vi "MotionProfileGenerator2.vi"(1 "MotionProfileGeneratorParameters":T1={"Trajectory Point Interval (ms)"=10, "Maximum Travel Speed (units/s)"=0.0, "Velocity Ramp Time (ms)"=0.0, "Acceleration Ramp Time (ms)"=1.0} {"Acceleration Ramp Time (ms)" min=1.0; "Velocity Ramp Time (ms)" min=1.0; "Maximum Travel Speed (units/s)" min=0.0; "Trajectory Point Interval (ms)" items=["TrajectoryDuration_0ms"=0, "TrajectoryDuration_5ms"=5, "TrajectoryDuration_10ms"=10, "TrajectoryDuration_20ms"=20, "TrajectoryDuration_30ms"=30, "TrajectoryDuration_40ms"=40, "TrajectoryDuration_50ms"=50, "TrajectoryDuration_100ms"=100]}, 2 "Starting Position (units)":dbl, 3 "Travel Distance (units)":dbl) -> (0 "Trajectory Points":T3[](array[typedef]) {"Time (ms)" items=["TrajectoryDuration_0ms"=0, "TrajectoryDuration_5ms"=5, "TrajectoryDuration_10ms"=10, "TrajectoryDuration_20ms"=20, "TrajectoryDuration_30ms"=30, "TrajectoryDuration_40ms"=40, "TrajectoryDuration_50ms"=50, "TrajectoryDuration_100ms"=100]})   [LabVIEW 2018, in "ArgosLib.lvlib"]
uses:
  ArgosLib.lvlib
  TypeDefs/TrajectoryPoint.ctl
  <vilib>/Rock Robotics/WPI/ThirdParty/Phoenix-LabVIEW/Motor Controller/Controls/CTRE_Phoenix_MotorControl_TrajectoryPointTimeDur.ctl
  TypeDefs/MotionProfileGeneratorParams.ctl
panel:
  out "Input":bool
  out "T4":dbl
  out "fl2":dbl
  out "fl1":dbl
  out "n":dbl
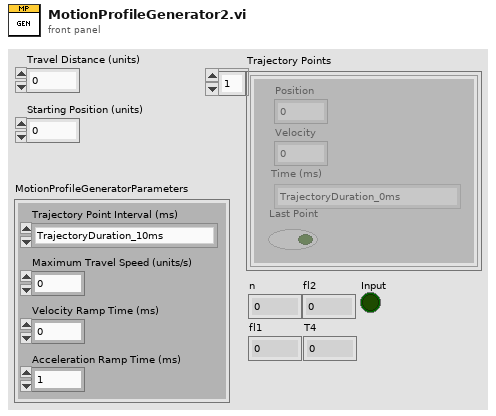
[diagram p1: front panel]
types:
  T1 = typedef "ArgosLib.lvlib/MotionProfileGeneratorParams.ctl" = cluster{"Trajectory Point Interval (ms)":T2, "Maximum Travel Speed (units/s)":dbl, "Velocity Ramp Time (ms)":dbl, "Acceleration Ramp Time (ms)":dbl}
  T2 = typedef "CTRE_Phoenix_MotorControl_TrajectoryPointTimeDur.ctl" = i32
  T3 = typedef "ArgosLib.lvlib/TrajectoryPoint.ctl" = cluster{"Position ":dbl, "Velocity ":dbl, "Time (ms)":T2, "Last Point":bool}
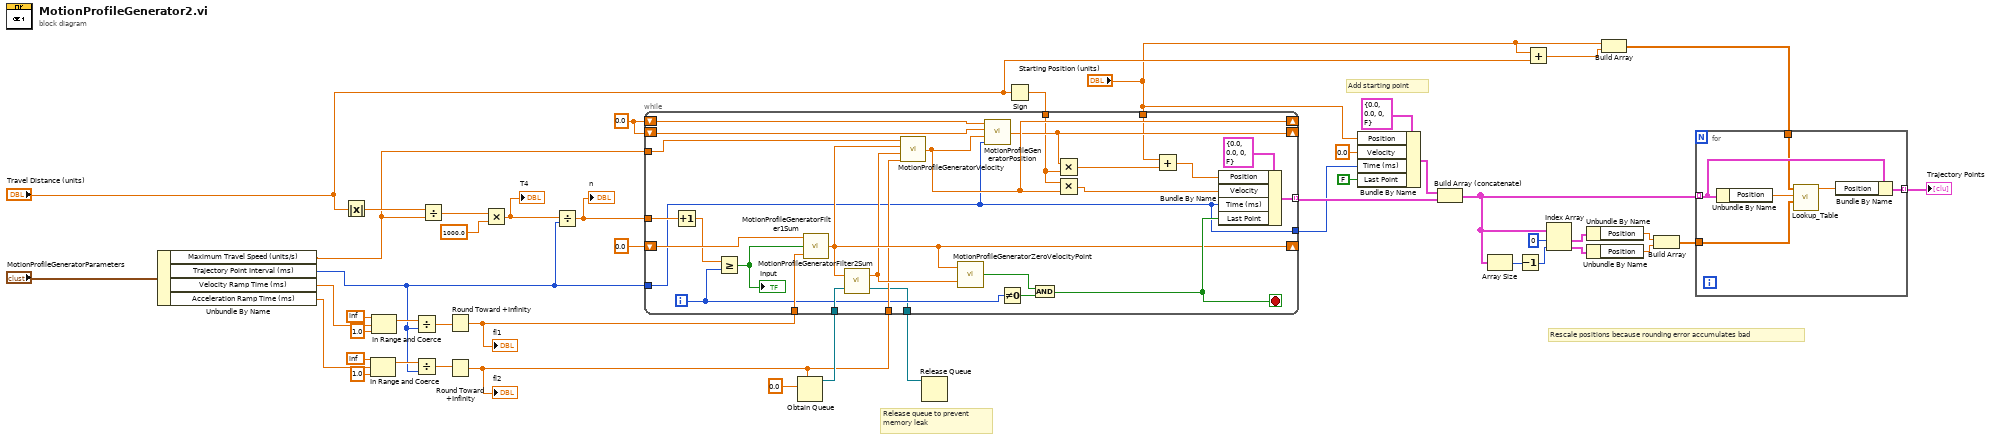
[diagram p0: block diagram]
diagram:
  w28 = 0.0
  # "Rescale positions because rounding error accumulates bad"
  # "Release queue to prevent\nmemory leak"
  # "Add starting point"
  n1 = Unbundle By Name("MotionProfileGeneratorParameters") -> ("Maximum Travel Speed (units/s)"=w15:dbl, "Trajectory Point Interval (ms)"=w25:T2, "Velocity Ramp Time (ms)"=w24:dbl, "Acceleration Ramp Time (ms)"=w23:dbl)
  n2 = Absolute Value(x="Travel Distance (units)") -> (abs(x)=w37:dbl)
  n3 = In Range and Coerce(upper limit=inf, x=w23, lower limit=1.0) -> (coerced(x)=w33:dbl)  [unwired: 1 out]
  n4 = In Range and Coerce(upper limit=inf, x=w24, lower limit=1.0) -> (coerced(x)=w34:dbl)  [unwired: 1 out]
  n5 = Divide(x=w34, y=w25) -> (x/y=w43:dbl)
  n6 = Divide(x=w33, y=w25) -> (x/y=w44:dbl)
  n7 = Divide(x=w37, y=w15) -> (x/y=w46:dbl)
  n8 = Round Toward +Infinity(x=w43) -> (ceil(x): smallest int >= x=w36:dbl)
  "fl1" <- w36
  n9 = Round Toward +Infinity(x=w44) -> (ceil(x): smallest int >= x=w35:dbl)
  "fl2" <- w35
  n10 = Multiply(x=w46, y=1000.0) -> (x*y=w42:dbl)
  "T4" <- w42
  n11 = Divide(x=w42, y=w25) -> (x/y=w41:dbl)
  "n" <- w41
  n12 = Obtain Queue(max queue size (-1, unlimited)=w35, element data type=0.0) -> (queue out=w38:refnum<queue>)  [unwired: 3 in, 2 out]
  n13 = Sign(1:"Travel Distance (units)") -> (0:w27:dbl)
  n14 = while {
    tunnel: w25 -> [w47]
    tunnel: w41 -> [w73]
    shift-right: [w62] -> _
    shift-left: 0.0 -> [w64]
    tunnel: w38 -> [w66]
    tunnel: [w70] -> w17 mode=indexing
    tunnel: w35 -> [w60]
    tunnel: w15 -> [w63]
    shift-right: [w55] -> _
    shift-left: w28 -> [w68]
    shift-right: [w53] -> _
    shift-left: w28 -> [w59]
    tunnel: w36 -> [w65]
    tunnel: w27 -> [w52]
    tunnel: [w49] -> w22
    tunnel: "Starting Position (units)" -> [w48]
    tunnel: [w47] -> w16
    i -> [w58]
    stop <- w69 stop-if-true
    n15 = Increment(x=w73) -> (x+1=w57:dbl)
    n16 = Greater Or Equal?(x=w57, y=w58) -> (x >= y?=w56:bool)
    "Input" <- w56
    n17 = call "MotionProfileGeneratorFilter1Sum.vi"("fl1"=w65, "Input"=w56, "Previous Filter1Sum"=w64) -> ("Filter1Sum"=w62:dbl)
    n18 = call "MotionProfileGeneratorFilter2Sum.vi"("Filter Queue"=w66, "Filter1Sum"=w62) -> ("queue out"=w49:refnum<queue>, "Filter2Sum"=w61:dbl)
    n19 = call "MotionProfileGeneratorVelocity.vi"("FL2"=w60, "filter2sum"=w61, "Filter1Sum"=w62, "Maximum Travel Speed (rps)"=w63) -> ("Velocity"=w55:dbl)
    n20 = call "MotionProfileGeneratorZeroVelocityPoint.vi"("Filter2Sum"=w61, "Filter1Sum"=w62) -> ("Zero Velocity"=w67:bool)
    n21 = call "MotionProfileGeneratorPosition.vi"("Trajectory Point Interval (ms)"=w47, "Velocity"=w55, "Previous Position"=w59, "Previous Velocity"=w68) -> ("Position"=w53:dbl)
    n22 = Not Equal To 0?(x=w58) -> (x != 0?=w72:bool)
    n23 = And(x=w67, y=w72) -> (x .and. y?=w69:bool)
    n24 = Multiply(x=w53, y=w52) -> (x*y=w51:dbl)
    n25 = Multiply(x=w52, y=w55) -> (x*y=w54:dbl)
    n26 = Add(x=w48, y=w51) -> (x+y=w50:dbl)
    n27 = Bundle By Name(cluster=T3 {"Position "=0.0, "Velocity "=0.0, "Time (ms)"=0, "Last Point"=FALSE} ("trajectory point"), "Position"=w50, "Velocity"=w54, "Time (ms)"=w47, "Last Point"=w69) -> (w70:T3)
  }
  n28 = Release Queue(queue=w22) -> ()  [unwired: 2 in, 3 out]
  n29 = Bundle By Name(cluster=T3 {"Position "=0.0, "Velocity "=0.0, "Time (ms)"=0, "Last Point"=FALSE} ("trajectory point"), "Position"="Starting Position (units)", "Velocity"=0.0, "Time (ms)"=w16, "Last Point"=FALSE) -> (w20:T3)
  n30 = Build Array (concatenate)(w20, w17) -> (w13:T3[])
  n31 = Array Size(array=w13) -> (size(s)=w12:i32)
  n32 = Decrement(x=w12) -> (x-1=w11:i32)
  n33 = Add(x="Starting Position (units)", y="Travel Distance (units)") -> (x+y=w3:dbl)
  n34 = Index Array(array=w13, index #1=0 ("index"), index #2=w11) -> (element #1=w9:T3, element #2=w8:T3)
  n35 = Unbundle By Name(w9) -> ("Position"=w7:dbl)
  n36 = Unbundle By Name(w8) -> ("Position"=w6:dbl)
  n37 = Build Array("Starting Position (units)", w3) -> (w2:dbl[])
  n38 = Build Array(w7, w6) -> (w1:dbl[])
  n39 = for {
    tunnel: w13 -> [w78] mode=indexing
    tunnel: [w76] -> w14 mode=indexing
    tunnel: w2 -> [w75]
    tunnel: w1 -> [w74]
    n40 = Unbundle By Name(w78) -> ("Position"=w79:dbl)
    n41 = call "Lookup_Table.vi"("Y_Array"=w75, "x_in"=w79, "X_Array"=w74) -> ("y_out"=w77:dbl)  [unwired: 6 in]
    n42 = Bundle By Name(cluster=w78, "Position"=w77) -> (w76:T3)
  }
  "Trajectory Points" <- w14
